vi "Translator.File.Read.Font.vi"(6 "Do not save font? (F)":bool, 8 "error in":errorcluster, 11 "Translation file":path=path "D:/PL_0125_Sapphire_Automation_branches/SOFTWARE_v1.1-Translation/settings/Translation-Chinese.ini") -> (0 "error out":errorcluster, 1 "font name":string="abcdefghijklmnopqrstuvwxyz", 2 "restart required?":bool)   [LabVIEW 2016]
uses:
  Translator.Global.vi
  <vilib>/Utility/config.llb/Read Key (String).vi
  <vilib>/Utility/config.llb/Write Key (String).vi
  <vilib>/Utility/config.llb/NI_LVConfig.lvlib
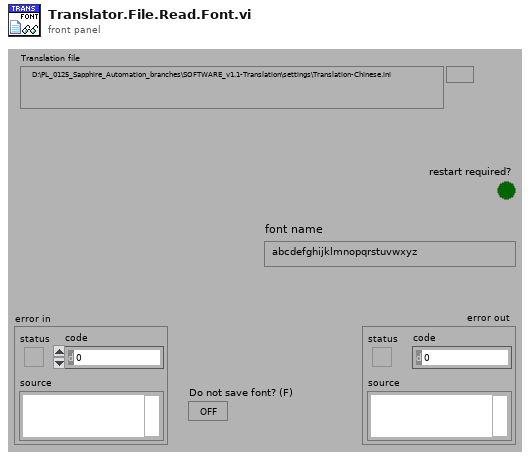
[diagram p1: front panel]
types:
  T1 = typedef "NI_LVConfig.lvlib/Config Data RefNum.ctl" = refnum<k1>
  T2 = enum32{"invalid app kind", "Development System", "Run Time System", "Student Edition", "Embedded LabVIEW", "Evaluation", "Custom"}
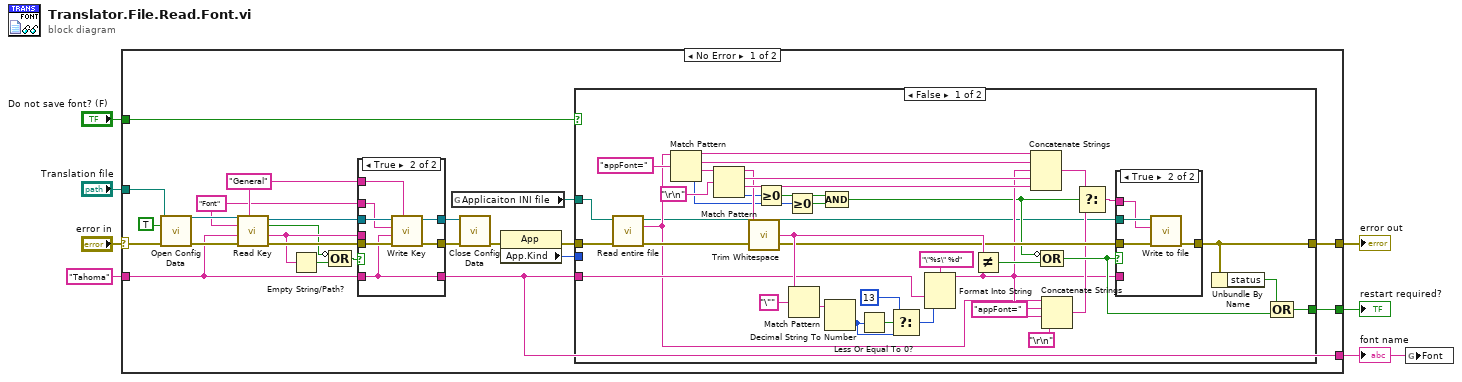
[diagram p0: block diagram]
diagram:
  n1 = case shown="No Error" "error in" {
    selector: "error in" -> [w20 w86]
    tunnel: [w12 w86] -> w7
    tunnel: "Translation file" -> [w21 _]
    tunnel: [w10 w85] -> w3
    tunnel: "Tahoma" ("default value") -> [w22 w85]
    tunnel: [w11 _] -> w2
    tunnel: "Do not save font? (F)" -> [w9 _]
    frame No Error {
      w23 = "Font" ("section")
      w24 = "General" ("section")
      n2 = call <vilib>:"Open Config Data.vi"("error in (no error)"=w20, "create file if necessary (T)"=TRUE, "configuration file path"=w21) -> ("error out"=w30:errorcluster, "refnum"=w29:T1)  [unwired: 6 in, 1 out]
      n3 = call-poly <vilib>:"Read Key.vi"("section"=w24, "error in (no error)"=w30, "default value"=w22, "key"=w23, "refnum"=w29) -> ("error out"=w28:errorcluster, "value"=w16:string, "found?"=w14:bool, "refnum out"=w25:T1)  [unwired: 3 in]
      n4 = Empty String/Path?(string/path=w16) -> (empty?=w15:bool)
      n5 = Compound Arithmetic op=OR(invert w14, w15) -> (w13:bool)
      n6 = case shown="True" w13 {
        tunnel: w28 -> [w77 w84]
        tunnel: [w77 w83] -> w27
        tunnel: [w76 w82] -> w26
        tunnel: w25 -> [w76 w81]
        tunnel: w24 -> [_ w80]
        tunnel: w23 -> [_ w79]
        tunnel: w16 -> [w75 _]
        tunnel: w22 -> [_ w78]
        tunnel: [w75 w78] -> w10
        frame False {
        }
        frame True {
          n7 = call-poly <vilib>:"Write Key.vi"("section"=w80, "error in (no error)"=w84, "value"=w78, "key"=w79, "refnum"=w81) -> ("error out"=w83:errorcluster, "refnum out"=w82:T1)  [unwired: 4 in, 1 out]
        }
      }
      n8 = global read "Translator.Global.vi" "Applicaiton INI file"() -> (w8:path)
      n9 = call <vilib>:"Close Config Data.vi"("error in (no error)"=w27, "refnum"=w26) -> ("error out"=w17:errorcluster)  [unwired: 8 in, 1 out]
      n10 = property class="App"(error in=w17) -> (error out=w18:errorcluster, "App.Kind"=w19:T2)  [unwired: 1 in, 1 out]
      n11 = case shown="False" w9 {
        tunnel: w19 -> [_ _]
        tunnel: w18 -> [w32 w74]
        tunnel: w10 -> [w49 _]
        tunnel: [w36 w74] -> w12
        tunnel: [w35 _] -> w11
        tunnel: w8 -> [w33 _]
        frame False {
          n12 = call "Read entire file.vi"("error in"=w32, "file"=w33) -> ("error out"=w56:errorcluster, "contents"=w43:string)  [unwired: 4 in]
          n13 = Match Pattern(string=w43, regular expression="appFont=" ("section")) -> (before substring=w54:string, match substring=w55:string, after substring=w51:string, offset past match=w41:i32)  [unwired: 1 in]
          n14 = Match Pattern(string=w51, regular expression="\r\n") -> (before substring=w50:string, match substring=w53:string, after substring=w52:string, offset past match=w42:i32)  [unwired: 1 in]
          n15 = call <vilib>:"Trim Whitespace.vi"("string"=w50) -> ("trimmed string"=w57:string)  [unwired: 1 in]
          n16 = Greater Or Equal To 0?(x=w42) -> (x >= 0?=w40:bool)
          n17 = Greater Or Equal To 0?(x=w41) -> (x >= 0?=w39:bool)
          n18 = Match Pattern(string=w57, regular expression="\"") -> (after substring=w58:string)  [unwired: 1 in, 3 out]
          n19 = Decimal String To Number(string=w58) -> (number=w63:i32)  [unwired: 2 in, 1 out]
          n20 = Compound Arithmetic op=AND(w40, w39) -> (w38:bool)
          n21 = Less Or Equal To 0?(x=w63) -> (x <= 0?=w64:bool)
          n22 = Select(t=13, s=w64, f=w63) -> (s? t:f=w62:i32)
          n23 = Format Into String(format string="\"%s\" %d", w49, w62) -> (resulting string=w45:string)  [unwired: 2 in, 1 out]
          n24 = Not Equal?(x=w57, y=w45) -> (x != y?=w68:bool)
          n25 = Concatenate Strings(w54, w55, w45, w53, w52) -> (w37:string)
          n26 = Compound Arithmetic op=OR(invert w38, w68) -> (w67:bool)
          n27 = Concatenate Strings(w43, "appFont=" ("string"), w45, "\r\n") -> (w46:string)
          n28 = Select(t=w37, s=w38, f=w46) -> (s? t:f=w44:string)
          n29 = case shown="True" w67 {
            tunnel: w56 -> [w69 w73]
            tunnel: [w69 w72] -> w36
            tunnel: w45 -> [_ _]
            tunnel: w33 -> [_ w71]
            tunnel: w44 -> [_ w70]
            frame False {
            }
            frame True {
              n30 = call "Write to file.vi"("error in"=w73, "addition"=w70, "file"=w71) -> ("error out"=w72:errorcluster)  [unwired: 8 in]
            }
          }
          n31 = Unbundle By Name(w36) -> ("status"=w34:bool)
          n32 = Compound Arithmetic op=OR(w34, w67) -> (w35:bool)
        }
        frame True {
        }
      }
    }
    frame Error {
    }
  }
  "error out" <- w7
  "font name" <- w3
  "restart required?" <- w2
  n33 = global write "Translator.Global.vi" "Font"(w3) -> ()
